vi "Get Front Panel Window Size.vi"(8 "error in":errorcluster, 11 "VI Ref":refnum<vi>) -> (0 "error out":errorcluster, 1 "FP:Window Size":cluster{"Width":i16, "Height":i16}, 2 "FP:Window Bounds":T1, 3 "VI Ref":refnum<vi>, 4 "FP:Panel Bounds":T1, 6 "FP:Panel Size":cluster{"Width":i16, "Height":i16})   [LabVIEW 2014]
doc: "Gets the FP bounds and calculates width and height."
uses:
  <vilib>/Utility/miscctls.llb/LVRectTypeDef.ctl
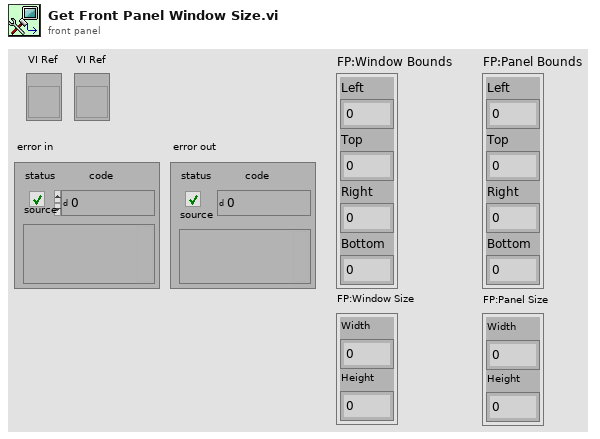
[diagram p1: front panel]
types:
  T1 = typedef "LVRectTypeDef.ctl" = cluster{"Left":i16, "Top":i16, "Right":i16, "Bottom":i16}
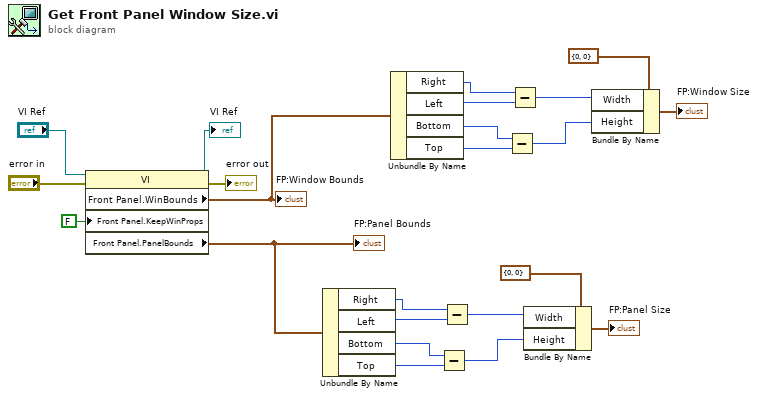
[diagram p0: block diagram]
diagram:
  n1 = property class="VI"(reference="VI Ref", error in="error in", "Front Panel.KeepWinProps"=FALSE ("Front Panel Window:Keep Window Proportions")) -> (reference out=→"VI Ref":refnum<vi>, error out=→"error out":errorcluster, "Front Panel.WinBounds"=w19:T1, "Front Panel.PanelBounds"=w2:T1)
  "FP:Window Bounds" <- w19
  "FP:Panel Bounds" <- w2
  n2 = Unbundle By Name(w2) -> ("Right"=w7:i16, "Left"=w8:i16, "Bottom"=w9:i16, "Top"=w1:i16)
  n3 = Unbundle By Name(w19) -> ("Right"=w14:i16, "Left"=w13:i16, "Bottom"=w12:i16, "Top"=w11:i16)
  n4 = Subtract(x=w9, y=w1) -> (x-y=w5:i16)
  n5 = Subtract(x=w7, y=w8) -> (x-y=w4:i16)
  n6 = Subtract(x=w12, y=w11) -> (x-y=w16:i16)
  n7 = Subtract(x=w14, y=w13) -> (x-y=w17:i16)
  n8 = Bundle By Name(cluster=cluster{"Width":i16, "Height":i16} {"Width"=0, "Height"=0}, "Width"=w4, "Height"=w5) -> (→"FP:Panel Size":cluster{"Width":i16, "Height":i16})
  n9 = Bundle By Name(cluster=cluster{"Width":i16, "Height":i16} {"Width"=0, "Height"=0}, "Width"=w17, "Height"=w16) -> (→"FP:Window Size":cluster{"Width":i16, "Height":i16})
